vi "test_Stop Monitor.vi"(8 "error in (no error)":errorcluster) -> (0 "error out":errorcluster, 3 "Data out":u64[](array[numeric])=[5631702913073631, 5629503829180420, 5629508124147720, 5629503829180426, 5629508124147722, 5629503829180426, 5629508124147722, 5629503829180426, 5629508124147722, 5631707147403291])   [LabVIEW 2016]
uses:
  Host/Typedefs/LV2G Operation.ctl
  Host/Typedefs/IO Buffer Operation.ctl
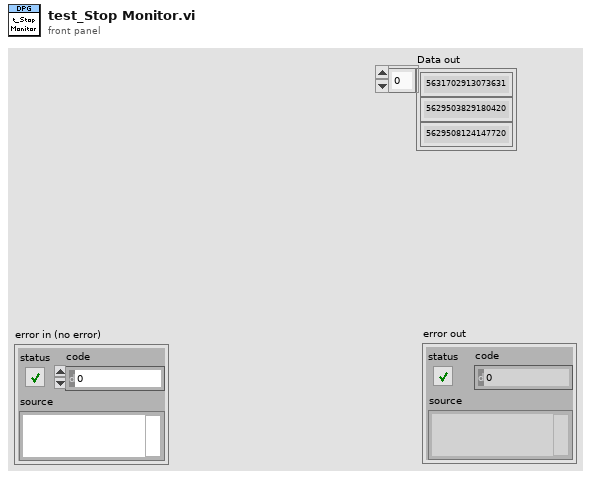
[diagram p1: front panel]
types:
  T1 = typedef "IO Buffer Operation.ctl" = enum16{"Initialize", "Write IO Data_Rd", "Read IO Data_Rd", "Write IO Data_Wr", "Read IO Data_Wr", "Write  IO Data_Dir", "Read  IO Data_Dir", "Write Host to Target FIFO", "Read Host to Target FIFO", "Write Target to Host FIFO", "Read Target to Host FIFO", "Write Monitor Enable?", "Read Monitor Enable?", "Close"}
  T2 = typedef "LV2G Operation.ctl" = enum16{"Initialize", "Set", "Get", "Close"}
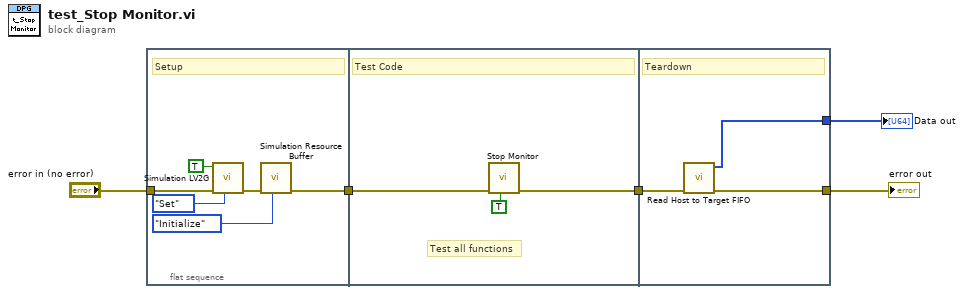
[diagram p0: block diagram]
diagram:
  n1 = flat-sequence {
    tunnel: "error in (no error)" -> [w11]
    tunnel: [w6] -> w5
    tunnel: w5 -> [w14]
    tunnel: [w13] -> w4
    tunnel: [w16] -> w2
    tunnel: w4 -> [w17]
    tunnel: [w15] -> w1
    frame #0 {
      # "Setup"
      n2 = call "Simulation LV2G.vi"("Operation (Get)"=LV2G_Operation."Set", "error in (no error)"=w11, "Simulation?"=TRUE) -> ("error out"=w8:errorcluster)  [unwired: 7 in, 1 out]
      n3 = call "Simulation Resource Buffer.vi"("IO Buffer Operation"=IO_Buffer_Operation."Initialize", "error in (no error)"=w8) -> ("error out"=w6:errorcluster)  [unwired: 7 in, 2 out]
    }
    frame #1 {
      # "Test all functions"
      # "Test Code"
      n4 = call "Stop Monitor.vi"("Write to FPGA(T)"=TRUE, "error in (no error)"=w14) -> ("error out"=w13:errorcluster)  [unwired: 8 in, 1 out]
    }
    frame #2 {
      # "Teardown"
      n5 = call "Read Host to Target FIFO.vi"("error in (no error)"=w17) -> ("error out"=w16:errorcluster, "Host to Target FIFO"=w15:u64[])  [unwired: 9 in]
    }
  }
  "error out" <- w2
  "Data out" <- w1
